vi "test No Missing Flag If All Options Are Present.vi"(8 "error in (no error)":errorcluster, 11 "TestCase in":refnum<class "Options Parsing Tests.lvclass">) -> (0 "error out":errorcluster, 3 "TestCase out":refnum<class "Options Parsing Tests.lvclass">)   [LabVIEW 2015, in "Options Parsing Tests.lvclass"]
uses:
  Options Parsing Tests.lvclass
  Argument Parser/Option Class/Option Configuration.ctl
  Argument Parser/Option Class/Argument Type.ctl
  <vilib>/addons/_JKI Toolkits/VI Tester/TestCase.llb/TestCase.lvclass
  Argument Parser/Option Set Class/Option Set.lvclass
  Argument Parser/Option Class/Option.lvclass
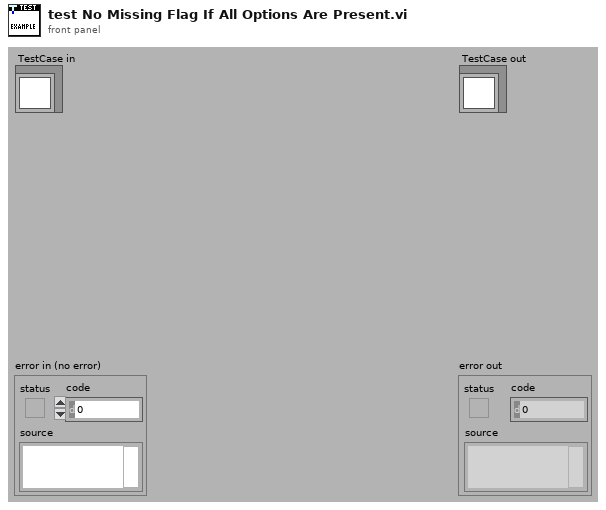
[diagram p1: front panel]
types:
  T1 = typedef "Option Parser.lvlib/Option.lvclass/Option Configuration.ctl" = cluster{"Option Type":T2, "Option Labels":string[], "Key":string, "Description":string, "Required":bool, "Default Value":string}
  T2 = typedef "Option Parser.lvlib/Option.lvclass/Argument Type.ctl" = enum16{"flag", "value"}
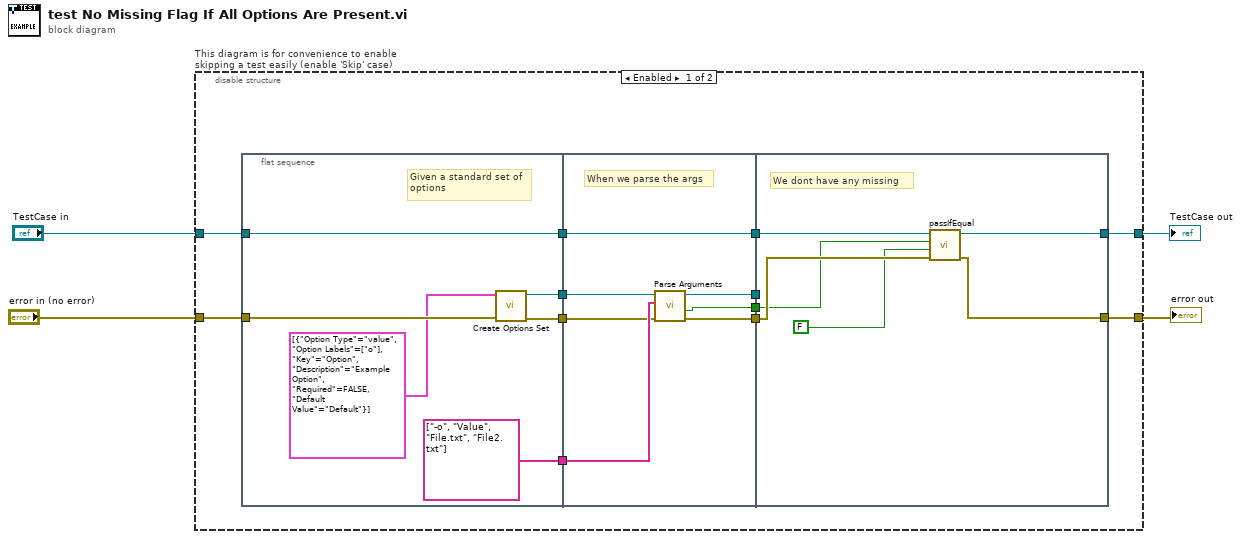
[diagram p0: block diagram]
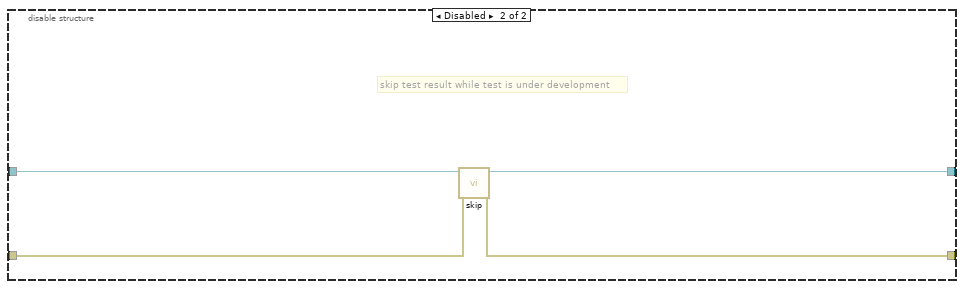
[diagram p2: hidden frame]
diagram:
  n1 = disable-structure "This diagram is for convenience to enable skipping a test easily (enable 'Skip' case)" shown="Enabled" {
    disable-tunnel: "TestCase in" -> [w8 w39]
    disable-tunnel: [w7 w37] -> w1
    disable-tunnel: [w6 w38] -> w3
    disable-tunnel: "error in (no error)" -> [w15 w36]
    frame Enabled {
      n2 = flat-sequence {
        tunnel: [string[] ["-o", "Value", "File.txt", "File2.txt"]] -> w16
        tunnel: w15 -> [w21]
        tunnel: [w20] -> w14
        tunnel: [w19] -> w13
        tunnel: [w18] -> w9
        tunnel: w8 -> [w18]
        tunnel: w16 -> [w29]
        tunnel: w14 -> [w28]
        tunnel: w13 -> [w27]
        tunnel: [w26] -> w12
        tunnel: [w25] -> w11
        tunnel: [w24] -> w10
        tunnel: w9 -> [w24]
        tunnel: [w23] -> w5
        tunnel: w12 -> [_]
        tunnel: w11 -> [w35]
        tunnel: w10 -> [w34]
        tunnel: [w32] -> w7
        tunnel: [w33] -> w6
        tunnel: w5 -> [w31]
        frame #0 {
          # "Given a standard set of\noptions"
          n3 = call "Create Options Set.vi"("error in (no error)"=w21, "Options"=T1[] [{"Option Type"=enum."value", "Option Labels"=["o"], "Key"="Option", "Description"="Example Option", "Required"=FALSE, "Default Value"="Default"}]) -> ("error out"=w20:errorcluster, "Option Set out"=w19:refnum<class "Option Set.lvclass">)  [unwired: 8 in]
        }
        frame #1 {
          # "When we parse the args"
          n4 = call "Parse Arguments.vi"("error in (no error)"=w28, "Arguments"=w29, "Option Set in"=w27) -> ("error out"=w25:errorcluster, "Missing Options"=w23:bool, "Option Set out"=w26:refnum<class "Option Set.lvclass">)  [unwired: 5 in, 1 out]
        }
        frame #2 {
          # "We dont have any missing"
          n5 = call-dynamic "passIfEqual.vi"("error in (no error)"=w35, "y"=FALSE ("Missing Options"), "x"=w31, "TestCase in"=w34) -> ("error out"=w33:errorcluster, "TestCase out"=w32:refnum<class "Options Parsing Tests.lvclass">)  [unwired: 6 in]
        }
      }
    }
    frame Disabled {
      # "skip test result while test is under development"
      n6 = call <vilib>:"skip.vi"("error in (no error)"=w36, "TestCase in"=w39) -> ("error out"=w38:errorcluster, "TestCase out"=w37:refnum<class "Options Parsing Tests.lvclass">)  [unwired: 8 in]
    }
  }
  "error out" <- w3
  "TestCase out" <- w1
